vi "Analog Ratio to Digital Switches.vi"(0 "Analog Ratio Input":dbl) -> (1 "High Output":bool, 2 "Low Output":bool)   [LabVIEW 2011]
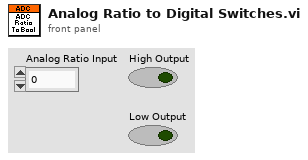
[diagram p1: front panel]
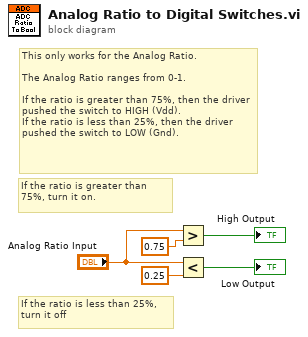
[diagram p0: block diagram]
diagram:
  # "This only works for the Analog Ratio.\n\nThe Analog Ratio ranges from 0-1.\n\nIf the ratio is greater than 75%, then the driver pushed the switch to HIGH (Vdd).\nIf the ratio is less than 25%, then the driver pushed the switch to LOW (Gnd)."
  # "If the ratio is less than 25%, turn it off"
  # "If the ratio is greater than 75%, turn it on."
  n1 = Greater?(x="Analog Ratio Input", y=0.75 ("Analog 2 (V)")) -> (0:→"High Output":bool)
  n2 = Less?(x="Analog Ratio Input", y=0.25) -> (x < y?=→"Low Output":bool)
